vi "delete.vi"() -> ()   [LabVIEW 2011]
panel:
  in  "Down?":bool
  in  "Lower Limit Switch":bool
  in  "Upper Limit Switch":bool
  out "Servo Close?":bool
  out "Output":dbl
  in  "Up":dbl=0.6
  in  "Down":dbl=-0.65
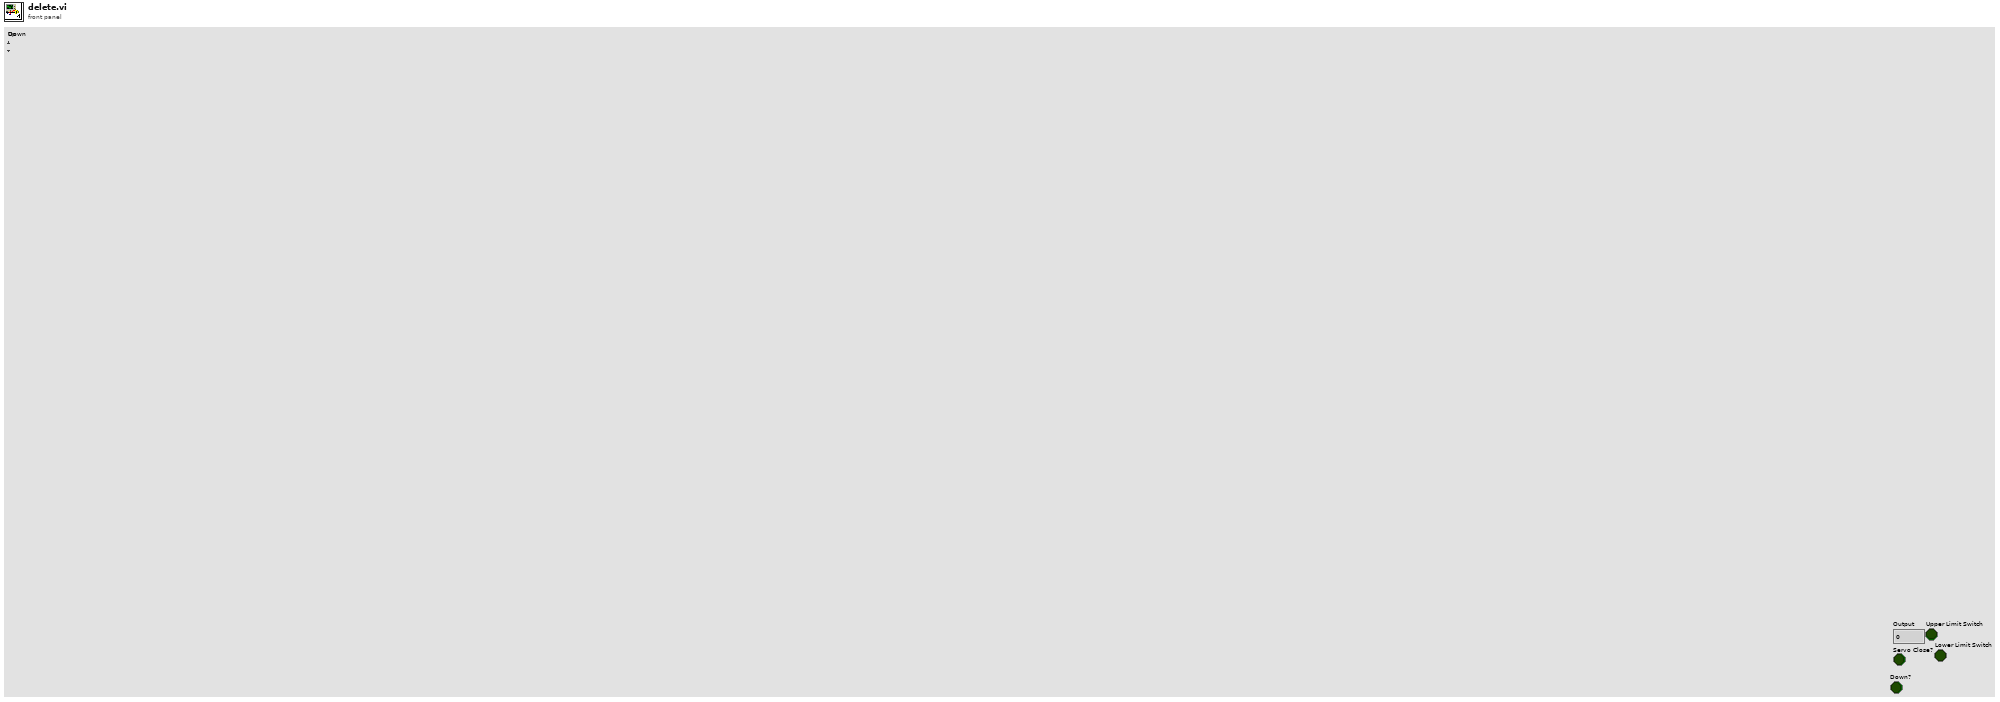
[diagram p1: front panel]
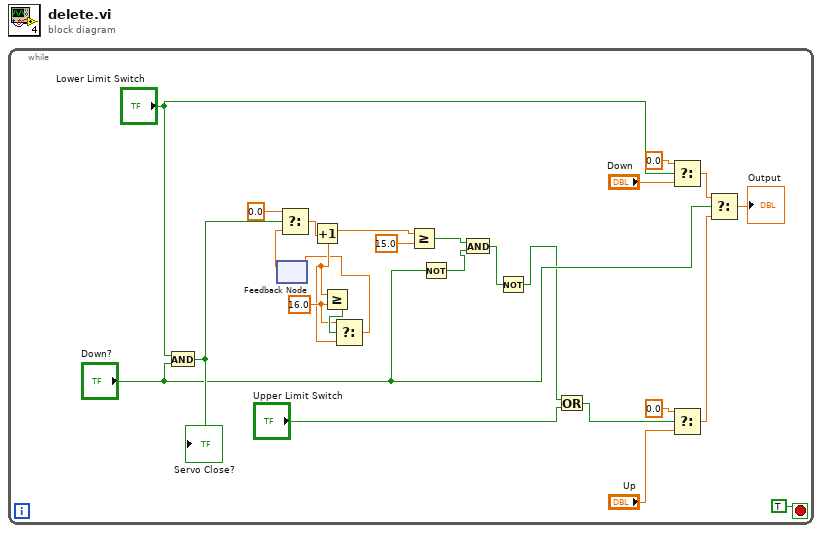
[diagram p0: block diagram]
diagram:
  n1 = while {
    stop <- TRUE stop-if-true
    w7 = 16.0 ("y")
    n2 = And(x="Lower Limit Switch", y="Down?") -> (x .and. y?=w16:bool)
    "Servo Close?" <- w16
    n3 = feedback #1() -> (w13:dbl)  [unwired: 1 in]
    n4 = Select(t=0.0, s=w16, f=w13) -> (s? t:f=w14:dbl)
    n5 = Increment(x=w14) -> (x+1=w6:dbl)
    n6 = Greater Or Equal?(x=w6, y=w7) -> (x >= y?=w8:bool)
    n7 = Select(t=w7, s=w8, f=w6) -> (s? t:f=w5:dbl)
    n8 = feedback-in #1(w5) -> ()
    n9 = Greater Or Equal?(x=w6, y=15.0) -> (x >= y?=w11:bool)
    n10 = Not(x="Down?") -> (.not. x?=w10:bool)
    n11 = And(x=w11, y=w10) -> (x .and. y?=w2:bool)
    n12 = Not(x=w2) -> (.not. x?=w1:bool)
    n13 = Or(x=w1, y="Upper Limit Switch") -> (x .or. y?=w3:bool)
    n14 = Select(t=0.0, s="Lower Limit Switch", f="Down") -> (s? t:f=w22:dbl)
    n15 = Select(t=0.0, s=w3, f="Up") -> (s? t:f=w23:dbl)
    n16 = Select(t=w22, s="Down?", f=w23) -> (s? t:f=→"Output":dbl)
  }
